vi "caseStructure.vi"() -> ()   [LabVIEW 2025]
panel:
  out "output":string
  in  "Enum":T1(ring)
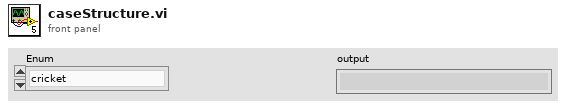
[diagram p1: front panel]
types:
  T1 = enum16{"cricket\n", "carrom\n", "chess\n", "badminton\n"}
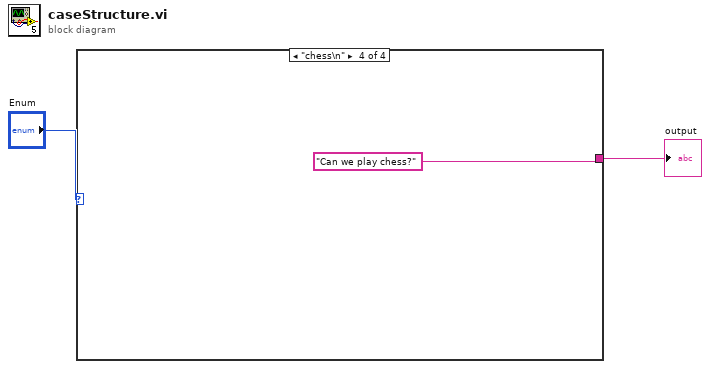
[diagram p0: block diagram]
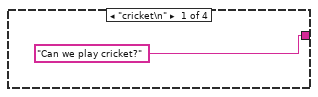
[diagram p2: hidden frame]
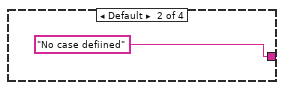
[diagram p3: hidden frame]
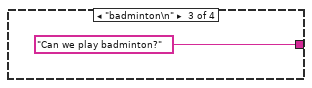
[diagram p4: hidden frame]
diagram:
  n1 = case shown="\"chess\\n\"" "Enum" {
    tunnel: ["Can we play cricket?" "No case defiined" "Can we play badminton?" "Can we play chess?"] -> w1
    frame "cricket\n" {
    }
    frame Default {
    }
    frame "badminton\n" {
    }
    frame "chess\n" {
    }
  }
  "output" <- w1
